vi "Modbus Test Timer.vi"(7 "Absolute Time":dbl format="%#.20f", 11 "Timing in":T1 {"Absolute Time" format="%<%H:%M:%S%3u>t"; "Display Time" format="%#.20f"; "Test Time Ref" format="%#.20f"; "Precondition Time Ref" format="%#.20f"; "First Call Time Ref" format="%#.20f"}) -> (3 "Timing Out":T1 {"Absolute Time" format="%<%H:%M:%S%3u>t"; "Display Time" format="%#.20f"; "Test Time Ref" format="%#.20f"; "Precondition Time Ref" format="%#.20f"; "First Call Time Ref" format="%#.20f"})   [LabVIEW 2020, in "Modbus.lvlib"]
uses:
  Modbus.lvlib
  Modbus Timing.ctl
  <vilib>/Utility/miscctls.llb/LVDateTimeRec.ctl
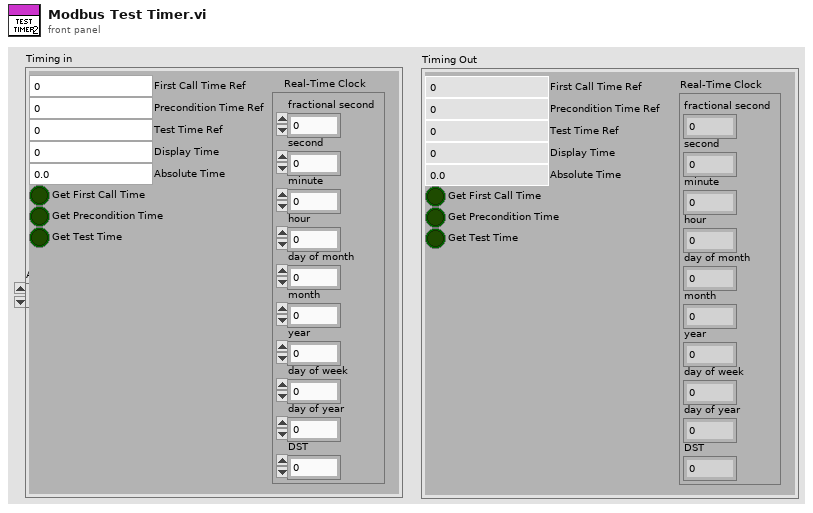
[diagram p1: front panel]
types:
  T1 = typedef "Modbus Timing.ctl" = cluster{"First Call Time Ref":dbl, "Precondition Time Ref":dbl, "Test Time Ref":dbl, "Get First Call Time":bool, "Get Precondition Time":bool, "Get Test Time":bool, "Display Time":dbl, "Real-Time Clock":T2, "Absolute Time":dbl}
  T2 = typedef "LVDateTimeRec.ctl" = cluster{"fractional second":dbl, "second":i32, "minute":i32, "hour":i32, "day of month":i32, "month":i32, "year":i32, "day of week":i32, "day of year":i32, "DST":i32}
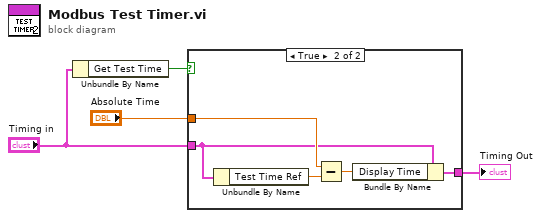
[diagram p0: block diagram]
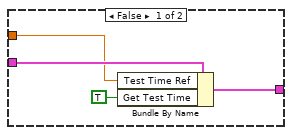
[diagram p2: hidden frame]
diagram:
  n1 = Unbundle By Name("Timing in") -> ("Get Test Time"=w2:bool)
  n2 = case shown="True" w2 {
    tunnel: [w8 w13] -> w1
    tunnel: "Timing in" -> [w7 w9]
    tunnel: "Absolute Time" -> [w5 w11]
    frame False {
      n3 = Bundle By Name(cluster=w7, "Test Time Ref"=w5, "Get Test Time"=TRUE) -> (w8:T1)
    }
    frame True {
      n4 = Unbundle By Name(w9) -> ("Test Time Ref"=w12:dbl)
      n5 = Subtract(x=w11, y=w12) -> (x-y=w10:dbl)
      n6 = Bundle By Name(cluster=w9, "Display Time"=w10) -> (w13:T1)
    }
  }
  "Timing Out" <- w1
